vi "SaveToHdf.vi"(5 "Input Data":u32[][](array[numeric]), 9 "Data folder path":path, 10 "String":string) -> ()   [LabVIEW 2015]
uses:
  <vilib>/UPVI/lvhdf5/file.llb/LVSWMR Type.ctl
  <vilib>/UPVI/lvhdf5/file.llb/LVH5F Operation.ctl
  <vilib>/Utility/miscctls.llb/LVRectTypeDef.ctl
  <vilib>/UPVI/lvhdf5/group.llb/H5G_obj_t.ctl
  <vilib>/UPVI/lvhdf5/dataset.llb/LVH5D Operation.ctl
  <vilib>/UPVI/lvhdf5/group.llb/OpenCreateGroup (String).vi
  <vilib>/UPVI/lvhdf5/utility.llb/Select HDF5 Dialog.vi
  <vilib>/UPVI/lvhdf5/utility.llb/Select HDF5 Dialog (Object Only).vi
  <vilib>/UPVI/lvhdf5/dataset.llb/Simple H5Dwrite (Variant).vi
  <vilib>/UPVI/lvhdf5/dataset.llb/Simple H5Dwrite.xnode
  <vilib>/UPVI/lvhdf5/library.llb/HDF5 Ref.ctl
  <vilib>/UPVI/lvhdf5/library.llb/HDF5 Ref.lvclass
  <vilib>/UPVI/lvhdf5/identifier.llb/Not an HDF5 Refnum Constant.vi
  <vilib>/Utility/error.llb/Error Cluster From Error Code.vi
  <vilib>/UPVI/lvhdf5/dataset.llb/OpenCreateReplace Dataset by Element Type.vi
  <vilib>/UPVI/lvhdf5/dataspace.llb/H5Sselect_hyperslab.vi
  <vilib>/UPVI/lvhdf5/dataset.llb/H5Dwrite (Variant).vi
  <vilib>/UPVI/lvhdf5/dataset.llb/H5Dget_space.vi
  <vilib>/UPVI/lvhdf5/attribute.llb/private/LVH5AwriteWDTAttrs.vi
  <vilib>/UPVI/lvhdf5/dataspace.llb/H5Sclose.vi
  <vilib>/UPVI/lvhdf5/dataset.llb/H5Dclose.vi
  <vilib>/UPVI/lvhdf5/utility.llb/Select HDF5 Dialog (File and Object).vi
panel:
  out "error out":errorcluster
  in  "error in":errorcluster
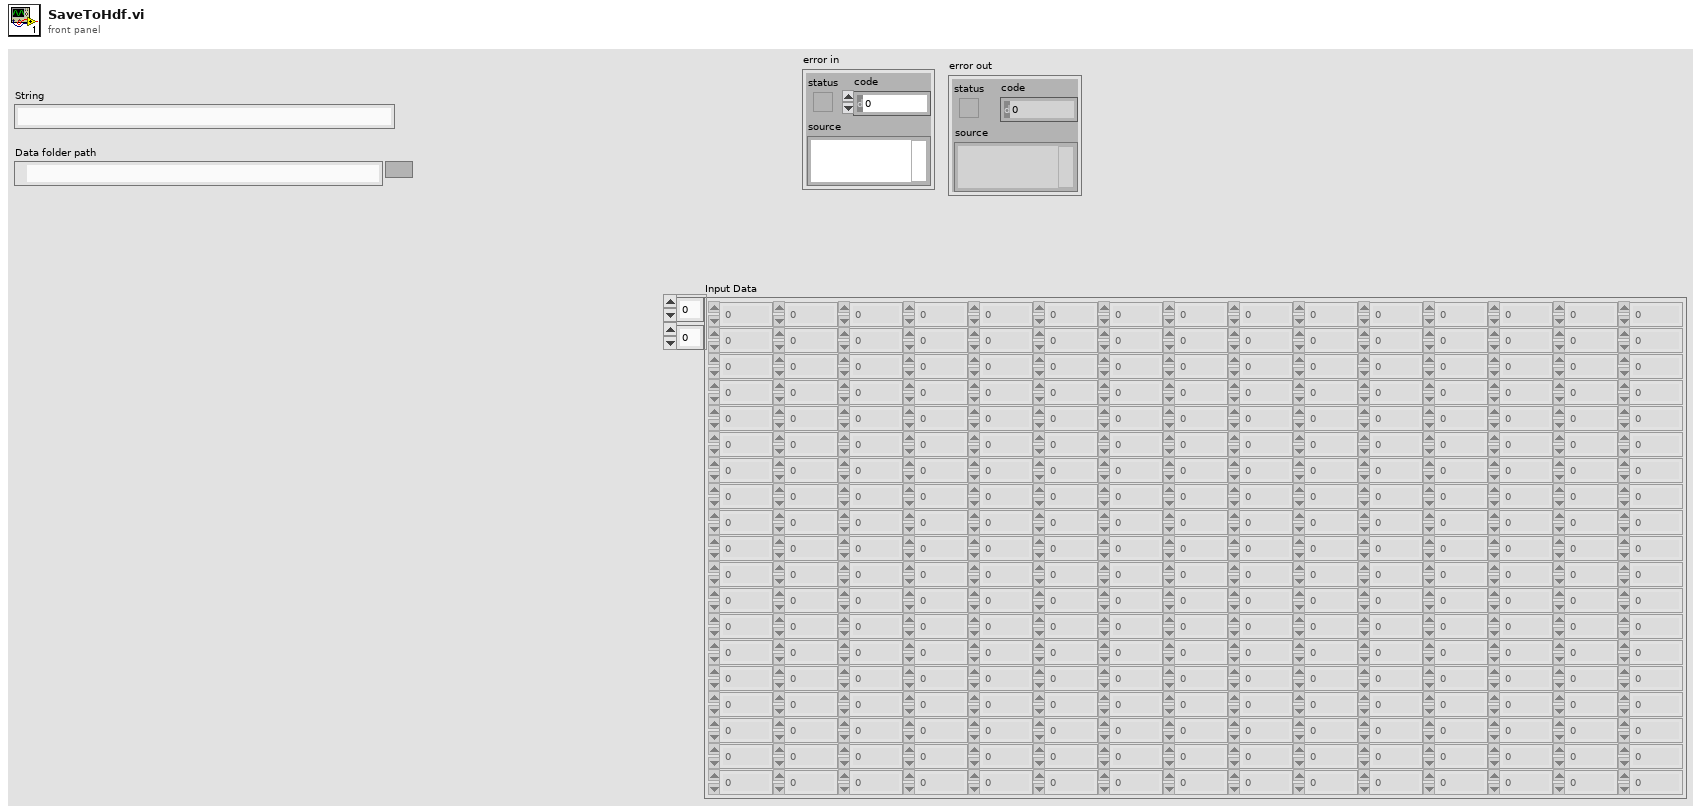
[diagram p1: front panel]
types:
  T1 = typedef "LVH5F Operation.ctl" = enum16{"open", "open or create", "create or replace", "create or replace (with confirmation)", "create", "open (read only)"}
  T2 = typedef "LVSWMR Type.ctl" = u32
  T3 = typedef "HDF5 Ref.ctl" = refnum<class "HDF5 Ref.lvclass">
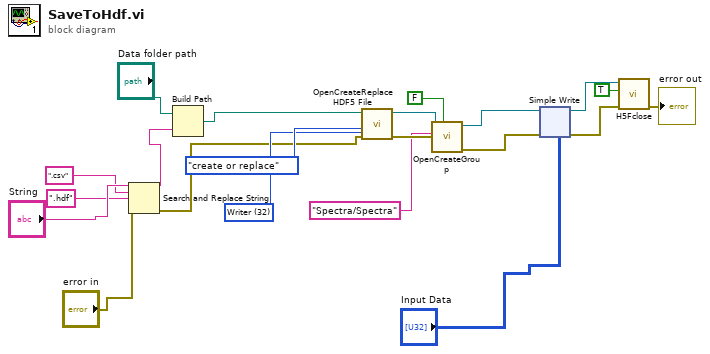
[diagram p0: block diagram]
diagram:
  w20 = T2 32 items=["None"=0, "Writer"=32, "Reader"=64] ("Single-write, multi-read")
  n1 = Search and Replace String(input string="String", search string=".csv" ("substring (\"\")"), replace string=".hdf" ("replace string (\"\")"), error in="error in") -> (result string=w5:string, error out=w4:errorcluster)  [unwired: 4 in, 2 out]
  n2 = Build Path(base path="Data folder path", name or relative path=w5) -> (appended path=w18:path)
  n3 = call <vilib>:"OpenCreateReplace HDF5 File.vi"("error in (no error)"=w4, "function (open or create)"=LVH5F_Operation."create or replace", "Single-write, multi-read"=w20, "path"=w18) -> ("error out"=w16:errorcluster, "HDF5 Ref out"=w17:T3)  [unwired: 4 in]
  n4 = call-poly <vilib>:"OpenCreateGroup.vi"("Create if not found (F)"=FALSE, "error in (no error)"=w16, "Group"="Spectra/Spectra", "HDF5 Ref"=w17) -> ("error out"=w13:errorcluster, "HDF5 Ref out"=w14:T3)  [unwired: 5 in, 1 out]
  n5 = xnode "Simple Write"("error in (no error)"=w13, "HDF5 Path or Ref"=w14, "Data"="Input Data") -> ("HDF5 Ref out"=w11:T3, "error out"=w10:errorcluster)  [unwired: 5 in, 1 out]
  n6 = call <vilib>:"H5Fclose.vi"("error in (no error)"=w10, "Close All Open Objects (T)"=TRUE, "HDF5 Ref"=w11) -> ("error out"=→"error out":errorcluster)  [unwired: 6 in]
